vi "Test JSON to Variant Errors.vi"() -> ()   [LabVIEW 2011]
uses:
  JSON Value/JSON Value.lvclass
  Variant JSON.lvlib
panel:
  out "Variant out":variant
  out "error out":errorcluster
  in  "JSON String 2":string
  out "data":T1
  in  "Test Cluster":T1={"T2"="test2", "T1"=456.789, "Nest"={"Enum"=enum."AAA", "NestNest"={"A"="Hi", "B"=2.0, "C"=1}}, "Test Array"=[456.789, 2.0, 3.0], "Boolean"=FALSE, "Time Stamp"=timestamp(0 s since 1904-01-01)}
  out "JSON String":string
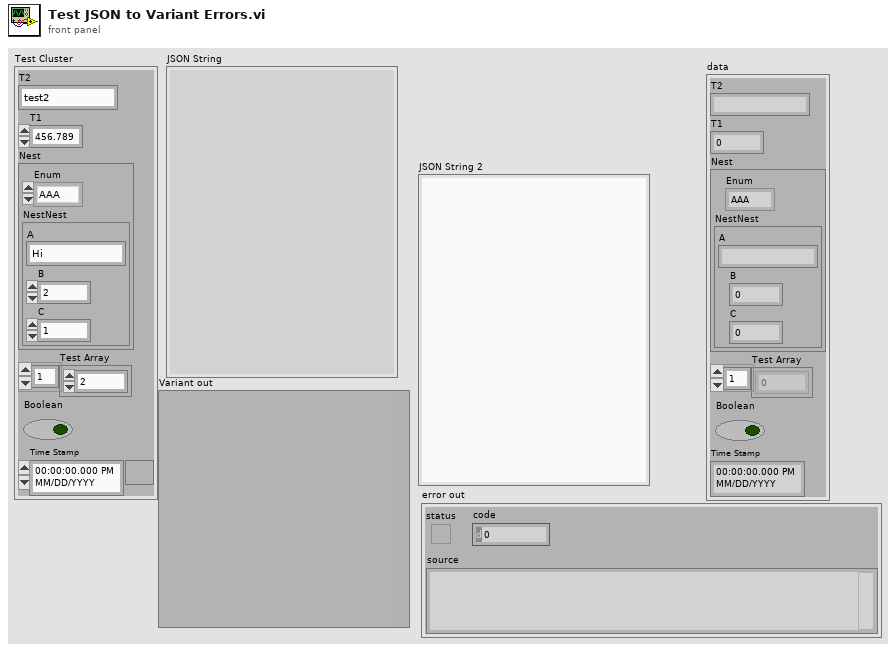
[diagram p1: front panel]
types:
  T1 = cluster{"T2":string, "T1":dbl, "Nest":cluster{"Enum":enum16{"AAA", "BBB", "CCC"}, "NestNest":cluster{"A":string, "B":dbl, "C":i16}}, "Test Array":dbl[], "Boolean":bool, "Time Stamp":timestamp}
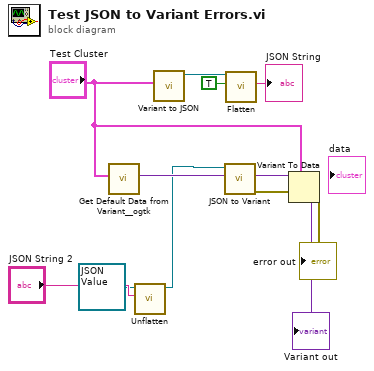
[diagram p0: block diagram]
diagram:
  n1 = call <userlib>:"Get Default Data from Variant__ogtk.vi"("Variant"="Test Cluster") -> ("Default VData"=w7:variant)  [unwired: 9 in, 1 out]
  n2 = call-dynamic "Unflatten.vi"("JSON stream"="JSON String 2", "JSON Value in"=refnum<class "JSON Value.lvclass"> refnum) -> ("JSON Value out"=w3:refnum<class "JSON Value.lvclass">)  [unwired: 6 in, 3 out]
  n3 = call "Variant to JSON.vi"("Variant"="Test Cluster") -> ("JSON Value out"=w2:refnum<class "JSON Value.lvclass">)  [unwired: 9 in, 1 out]
  n4 = call "JSON to Variant.vi"("Variant (Data Type)"=w7, "JSON Value"=w3) -> ("error out"=→"error out":errorcluster, "Variant out"=w8:variant)  [unwired: 8 in]
  "Variant out" <- w8
  n5 = call-dynamic "Flatten.vi"("Pretty Print?"=TRUE, "JSON Value in"=w2) -> ("String"=→"JSON String":string)  [unwired: 8 in, 1 out]
  n6 = Variant To Data(type="Test Cluster", Variant=w8) -> ()  [unwired: 1 in, 2 out]
